vi "Area.vi"(8 "error in (no error)":errorcluster, 11 "Proto in":refnum<class "Proto.lvclass">) -> (0 "error out":errorcluster, 2 "Area":u64, 3 "Proto out":refnum<class "Proto.lvclass">)   [LabVIEW 2021, in "Proto.lvclass"]
uses:
  Proto.lvclass
  Proto.lvclass/Proto.ctl
panel:
  out "Intensity Graph 4":i16[][](graph)
  out "Intensity Graph 3":i16[][](graph)
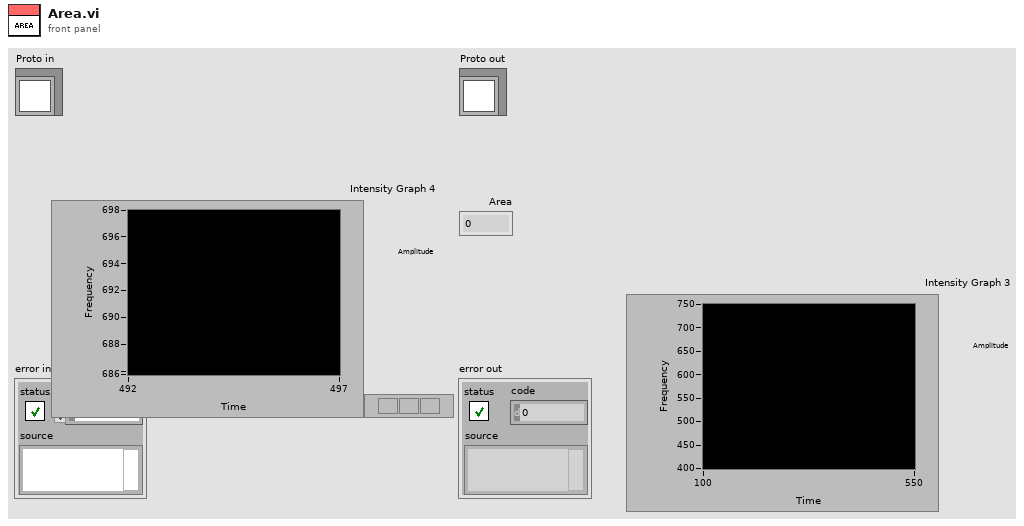
[diagram p1: front panel]
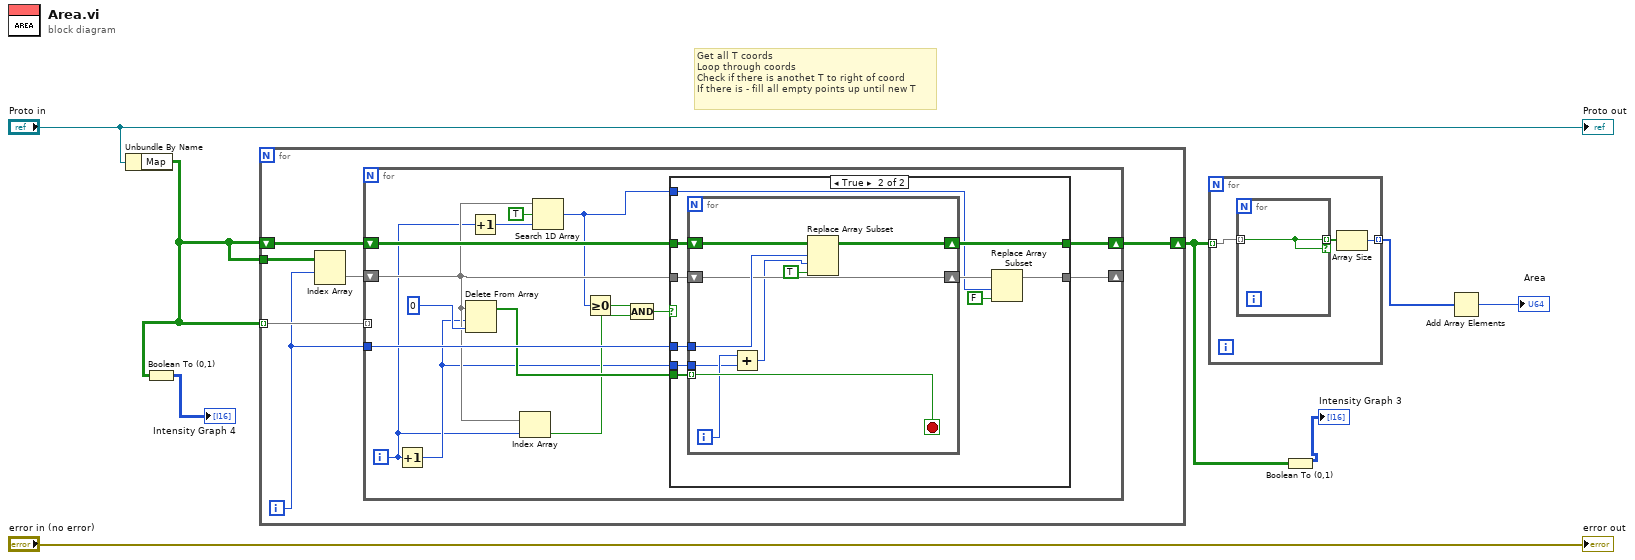
[diagram p0: block diagram]
diagram:
  # "Get all T coords\nLoop through coords\nCheck if there is anothet T to right of coord\nIf there is - fill all empty points up until new T"
  n1 = Unbundle By Name("Proto in") -> ("Map"=w3:bool[][])
  n2 = Boolean To (0,1)(Boolean=w3) -> (0, 1=→"Intensity Graph 4":i16[][])
  n3 = for {
    tunnel: w3 -> [w14] mode=indexing
    shift-right: [w13] -> w5
    shift-left: w3 -> [w12]
    tunnel: w3 -> [w9]
    i -> [w10]
    n4 = Index Array(array=w9, index (row)=w10) -> (element=w11:bool[])  [unwired: 1 in]
    n5 = for {
      tunnel: w14 -> [_] mode=indexing
      shift-right: [w27] -> w13
      shift-left: w12 -> [w28]
      tunnel: w10 -> [w26]
      shift-right: [w22] -> _
      shift-left: w11 -> [w21]
      i -> [w15]
      n6 = Increment(x=w15) -> (x+1=w16:i32)
      n7 = Delete From Array(array=w21, length=w16, index=0) -> (array with subset deleted=w24:bool[])  [unwired: 1 out]
      n8 = Increment(x=w15) -> (x+1=w17:i32)
      n9 = Index Array(array=w21, index=w15) -> (element=w23:bool)
      n10 = Search 1D Array(1D array=w21, element=TRUE, start index (0)=w17) -> (index of element=w18:i32)
      n11 = Greater Or Equal To 0?(x=w18) -> (x >= 0?=w19:bool)
      n12 = Compound Arithmetic op=AND(w19, w23) -> (w25:bool)
      n13 = case shown="True" w25 {
        tunnel: w28 -> [w31 w41]
        tunnel: [w31 w40] -> w27
        tunnel: w16 -> [_ w39]
        tunnel: w26 -> [_ w38]
        tunnel: w24 -> [_ w37]
        tunnel: [w30 w34] -> w22
        tunnel: w21 -> [w30 w36]
        tunnel: w18 -> [_ w33]
        frame False {
        }
        frame True {
          n14 = for {
            tunnel: w37 -> [w49] mode=indexing
            shift-right: [w48] -> w40
            shift-left: w41 -> [w50]
            tunnel: w39 -> [w46]
            tunnel: w38 -> [w45]
            shift-right: [w43] -> w35
            shift-left: w36 -> [w43]
            i -> [w47]
            stop <- w49 stop-if-true
            n15 = Add(x=w47, y=w46) -> (x+y=w42:i32)
            n16 = Replace Array Subset(array=w50, new element=TRUE ("new element/subarray"), index (row)=w45, index (col)=w42) -> (w48:bool[][])
          }
          n17 = Replace Array Subset(array=w35, new element=FALSE ("new element/subarray"), index=w33) -> (w34:bool[])
        }
      }
    }
  }
  n18 = for {
    tunnel: w5 -> [w52] mode=indexing
    tunnel: [w51] -> w6 mode=indexing
    n19 = for {
      tunnel: [w54] -> w53 mode=indexing if=w54
      tunnel: w52 -> [w54] mode=indexing
    }
    n20 = Array Size(array=w53) -> (size(s)=w51:i32)
  }
  n21 = Boolean To (0,1)(Boolean=w5) -> (0, 1=→"Intensity Graph 3":i16[][])
  n22 = Add Array Elements(numeric array=w6) -> (sum=→"Area":i32)
  "error out" <- "error in (no error)"
  "Proto out" <- "Proto in"
